vi "Read Color.vi"(8 "error in (no error)":errorcluster, 11 "CircleShape in":refnum<class "CircleShape.lvclass">) -> (0 "error out":errorcluster, 2 "Color out":u32(colorbox), 3 "CircleShape out":refnum<class "CircleShape.lvclass">)   [LabVIEW 2022 SP3, in "CircleShape.lvclass"]
uses:
  CircleShape.lvclass
  CircleShape.lvclass/CircleShape.ctl
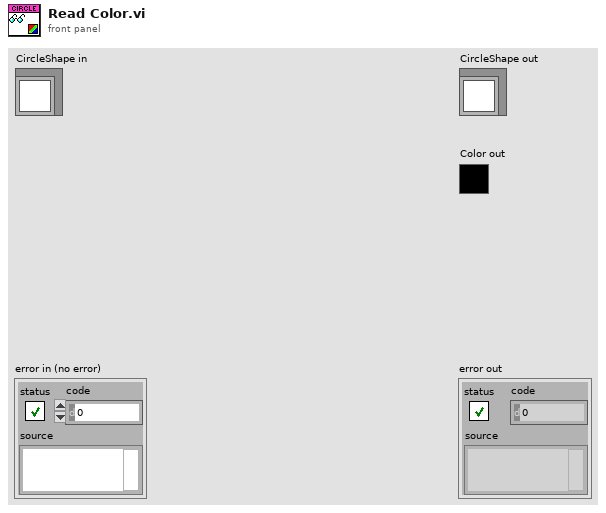
[diagram p1: front panel]
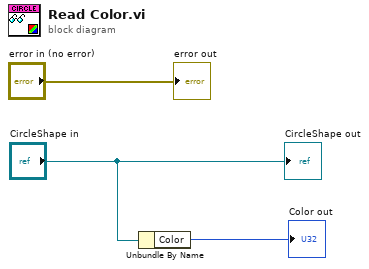
[diagram p0: block diagram]
diagram:
  n1 = Unbundle By Name("CircleShape in") -> ("Color"=→"Color out":u32)
  "error out" <- "error in (no error)"
  "CircleShape out" <- "CircleShape in"
